vi "Holo Size SLM.vi"() -> (8 "data":i32)   [LabVIEW 2014]
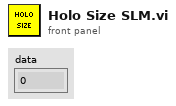
[diagram p1: front panel]
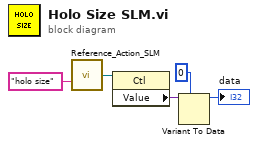
[diagram p0: block diagram]
diagram:
  n1 = call "Reference_Action_SLM.vi"("Control Name"="holo size") -> ("Ref OUT"=w4:refnum<vi>)  [unwired: 12 in, 2 out]
  n2 = property class="Ctl"(reference=w4) -> ("Value"=w3:variant)  [unwired: 1 in, 2 out]
  n3 = Variant To Data(type=0, Variant=w3) -> (data=→"data":i32)  [unwired: 1 in, 1 out]
